vi "Count Variations.vi"(10 "Array":i64[](array[numeric]), 11 "unsigned byte array":u8[](array[numeric])) -> (3 "Numeric":i64)   [LabVIEW 2021]
uses:
  <userlib>/_OpenG.lib/array/array.llb/Search 1D Array (U8)__ogtk.vi
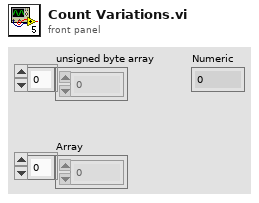
[diagram p1: front panel]
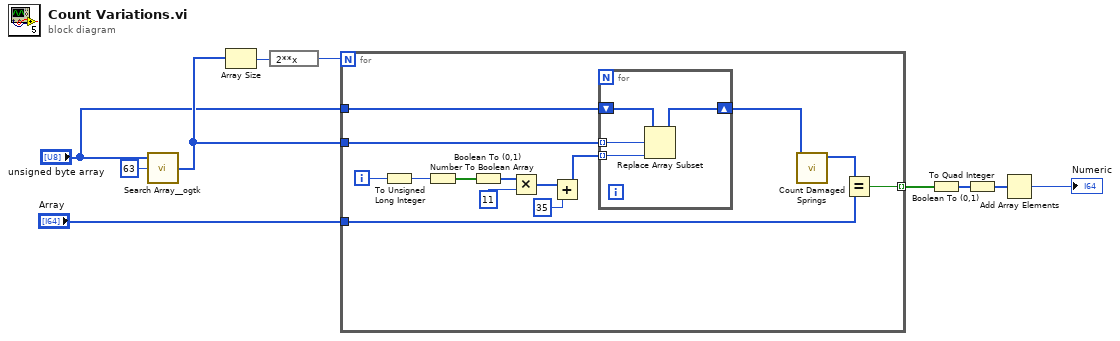
[diagram p0: block diagram]
diagram:
  n1 = call-poly <userlib>:"Search Array__ogtk.vi"("Array"="unsigned byte array", "Element Data"=u8 63) -> ("Indices of Elements"=w10:i32[])  [unwired: 7 in]
  n2 = Array Size(array=w10) -> (size(s)=w7:i32)
  n3 = expression code="2**x"(w7) -> (w8:i32)
  n4 = for {
    N: w8 -> [_]
    tunnel: "Array" -> [w23]
    tunnel: [w22] -> w2 mode=indexing
    tunnel: "unsigned byte array" -> [w15]
    tunnel: w10 -> [w14]
    i -> [w16]
    n5 = To Unsigned Long Integer(number=w16) -> (unsigned 32bit integer=w12:u32)
    n6 = Number To Boolean Array(number=w12) -> (Boolean array=w21:bool[])
    n7 = Boolean To (0,1)(Boolean=w21) -> (0, 1=w20:i16[])
    n8 = Multiply(x=w20, y=u8 11) -> (x*y=w18:i16[])
    n9 = Add(x=w18, y=u8 35) -> (x+y=w13:i16[])
    n10 = for {
      shift-right: [w25] -> w11
      shift-left: w15 -> [w27]
      tunnel: w14 -> [w28] mode=indexing
      tunnel: w13 -> [w26] mode=indexing
      n11 = Replace Array Subset(array=w27, new element=w26, index=w28) -> (w25:u8[])
    }
    n12 = call "Count Damaged Springs.vi"("Record In"=w11) -> ("Count Out"=w24:i64[])  [unwired: 10 in]
    n13 = Equal?(x=w24, y=w23) -> (x = y?=w22:bool)
  }
  n14 = Boolean To (0,1)(Boolean=w2) -> (0, 1=w3:i16[])
  n15 = To Quad Integer(1:w3) -> (0:w5:i64[])
  n16 = Add Array Elements(numeric array=w5) -> (sum=→"Numeric":i64)
